vi "init.vi"(8 "error in (no error)":errorcluster, 11 "bike in":refnum<class "bike.lvclass">) -> (0 "error out":errorcluster, 3 "bike out":refnum<class "bike.lvclass">)   [LabVIEW 2011, in "bike.lvclass"]
uses:
  bike.lvclass
  genericVehicle/vehicleGeneric.lvclass
  bike.lvclass/bike.ctl
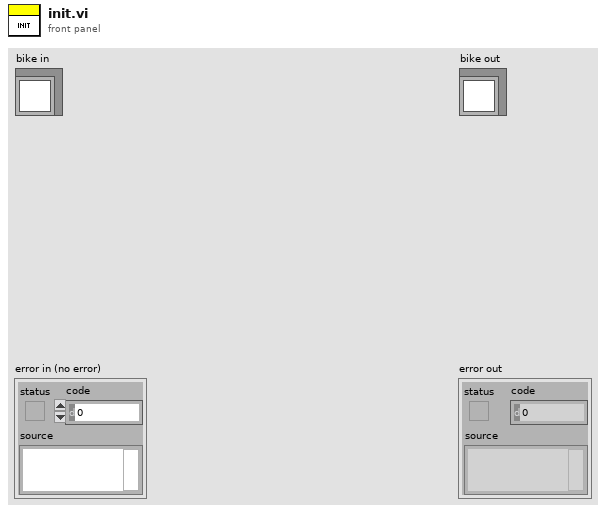
[diagram p1: front panel]
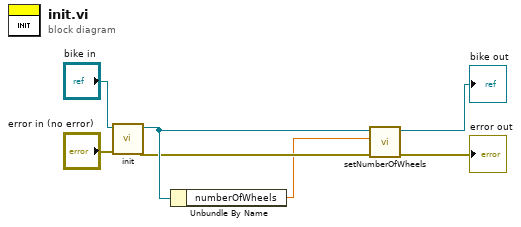
[diagram p0: block diagram]
diagram:
  n1 = call-parent "init.vi"("error in (no error)"="error in (no error)", "vehicleGeneric in"="bike in") -> ("error out"=w4:errorcluster, "vehicleGeneric out"=w5:refnum<class "bike.lvclass">)  [unwired: 8 in]
  n2 = Unbundle By Name(w5) -> ("numberOfWheels"=w1:dbl)
  n3 = call-dynamic "setNumberOfWheels.vi"("error in (no error)"=w4, "numberOfWheels"=w1, "vehicleGeneric in"=w5) -> ("error out"=→"error out":errorcluster, "vehicleGeneric out"=→"bike out":refnum<class "bike.lvclass">)  [unwired: 7 in]
